vi "Read Camera Setup.vi"(8 "error in (no error)":errorcluster, 10 "String Camera Setup":string="Acquisition Mode // 1\rRead Mode // 0\rTrigger // 0\rConventional/EM // 1\rShutter Mode // 2\rShutter TTL // 0\rTime to open Shutter // 50\rTime to close Shutter // 50\rExposure time // 0\rReadout Rate // 0\rVShift Speed // 0\rPre amp // 1\rInitial line // 1\rInitial column // 1\rFinal column // 1\rFinal line // 1\rhbin // 1\rvbin // 1\rTemperature // 20\rCooler ON/OFF // 0\rFITS Format // 0\rtiff position // 1\rTiff Type // 0\rImage Format // 0\r", 11 "Construct String Setup Cam in":refnum<class "Construct String Setup Cam.lvclass">) -> (0 "error out":errorcluster, 2 "Camera Setup":T1={"Acquisition Mode"=1, "Read Mode"=4, "Trigger"=0, "Conventional/EM"=0, "Shutter Mode"=2, "Shutter TTL"=0, "Time to open Shutter"=50, "Time to close Shutter"=50, "Exposure time"=0.0, "Readout Rate"=0, "VShift Speed"=0, "Pre amp"=0, "Initial line"=1, "Initial column"=1, "Final column"=1024, "Final line"=1024, "hbin"=1, "vbin"=1, "Temperature"=20.0, "Cooler ON/OFF"=0, "FITS Format"=0, "tiff position"=1, "Tiff Type"=0, "Image Format"="", "Image Path"=""} {"Tiff Type" items=["8-bit", "16-bit", "Color"]; "FITS Format" items=["Unsigned 16", "Unsigned 32", "Signed 16", "Signed 32", "Float"]; "Cooler ON/OFF" items=["Cooler OFF", "Cooler ON"]; "Shutter TTL" items=["TTL Low", "TTL High"]; "Shutter Mode" items=["Fully Auto", "OPEN", "CLOSED"]; "Conventional/EM" items=["Conventional", "EM Gain"]; "Trigger" items=["Internal", "External", "N/A", "N/A", "N/A", "N/A", "External Start", "External Exposure (bulb)", "N/A", "External FVB EM", "Software", "N/A", "External Charge Shifting"]; "Read Mode" items=["Full Vertical Binning", "Multi-Track", "Random-Track", "Single-Track", "Image"]; "Acquisition Mode" items=["RESERVED", "Single Scan", "Accumulate", "Kinetics", "Fast Kinetics", "Run Til Abort", "RESERVED", "RESERVED", "RESERVED", "RESERVED", "Time Delayed Integration"]}, 3 "Construct String Setup Cam out":refnum<class "Construct String Setup Cam.lvclass">)   [LabVIEW 2018, in "Construct String Setup Cam.lvclass"]
doc: "Este VI recebe uma string contendo a configuração da câmera e retorna um cluster com as informações da configuração."
uses:
  Construct String Setup Cam.lvclass
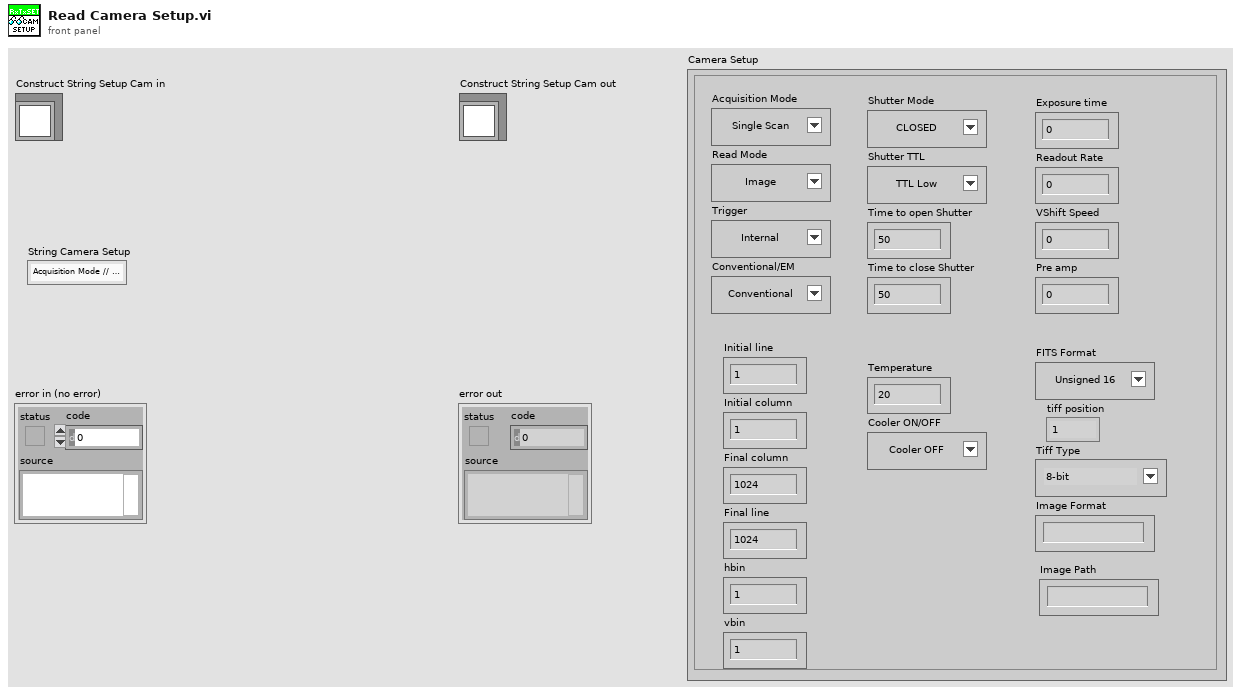
[diagram p1: front panel]
types:
  T1 = cluster{"Acquisition Mode":u16, "Read Mode":u16, "Trigger":u16, "Conventional/EM":u16, "Shutter Mode":u16, "Shutter TTL":u16, "Time to open Shutter":u16, "Time to close Shutter":u16, "Exposure time":dbl, "Readout Rate":u16, "VShift Speed":u16, "Pre amp":u16, "Initial line":u16, "Initial column":u16, "Final column":u32, "Final line":u32, "hbin":u16, "vbin":u16, "Temperature":dbl, "Cooler ON/OFF":u16, "FITS Format":u16, "tiff position":u16, "Tiff Type":u16, "Image Format":string, "Image Path":string}
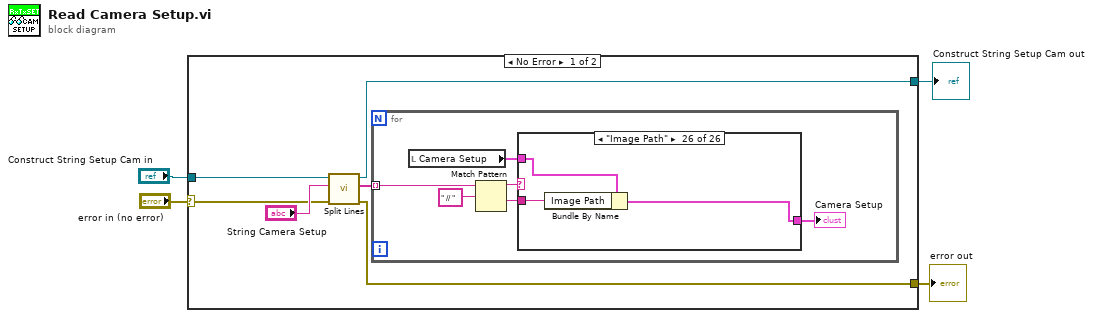
[diagram p0: block diagram]
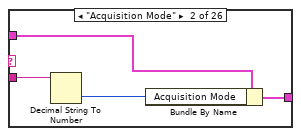
[diagram p3: hidden frame]
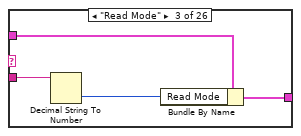
[diagram p4: hidden frame]
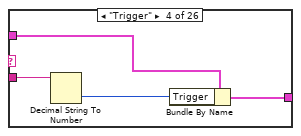
[diagram p5: hidden frame]
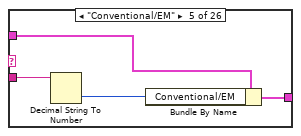
[diagram p6: hidden frame]
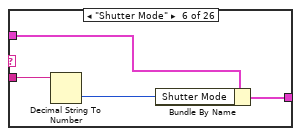
[diagram p7: hidden frame]
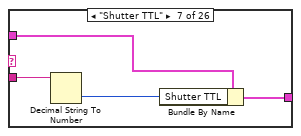
[diagram p8: hidden frame]
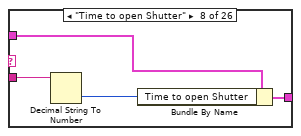
[diagram p9: hidden frame]
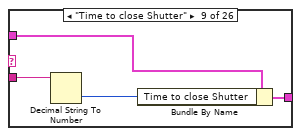
[diagram p10: hidden frame]
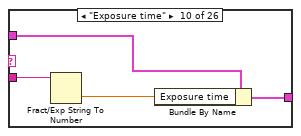
[diagram p11: hidden frame]
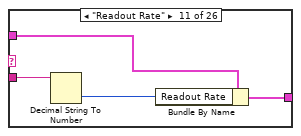
[diagram p12: hidden frame]
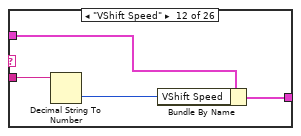
[diagram p13: hidden frame]
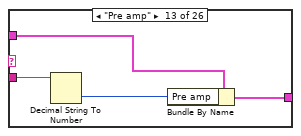
[diagram p14: hidden frame]
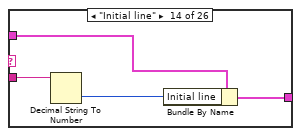
[diagram p15: hidden frame]
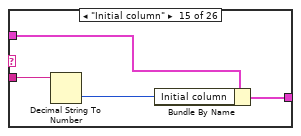
[diagram p16: hidden frame]
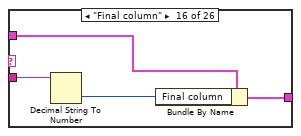
[diagram p17: hidden frame]
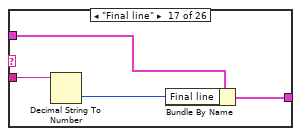
[diagram p18: hidden frame]
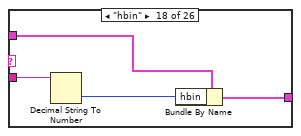
[diagram p19: hidden frame]
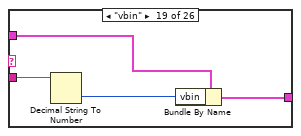
[diagram p20: hidden frame]
diagram:
  n1 = case shown="No Error" "error in (no error)" {
    selector: "error in (no error)" -> [w9 w116]
    tunnel: [w8 w116] -> w3
    tunnel: [w6 w117] -> w1
    tunnel: "Construct String Setup Cam in" -> [w7 w117]
    frame No Error {
      n2 = call "Split Lines.vi"("error in (no error)"=w9, "spreadsheet string"="String Camera Setup", "Construct String Setup Cam in"=w7) -> ("error out"=w8:errorcluster, "array"=w5:string[], "Construct String Setup Cam out"=w6:refnum<class "Construct String Setup Cam.lvclass">)  [unwired: 6 in]
      n3 = for {
        tunnel: w5 -> [w16] mode=indexing
        n4 = local read "Camera Setup"() -> (w12:T1)
        n5 = Match Pattern(string=w16, regular expression=" // ") -> (before substring=w14:string, after substring=w13:string)  [unwired: 1 in, 2 out]
        n6 = case shown="\"Image Path\"" w14 {
          tunnel: w13 -> [_ w19 w22 w26 w30 w34 w38 w42 w46 w50 w54 w58 w62 w66 w70 w74 w78 w82 w86 w90 w94 w98 w102 w106 w110 w113]
          tunnel: w12 -> [w17 w21 w24 w28 w32 w36 w40 w44 w48 w52 w56 w60 w64 w68 w72 w76 w80 w84 w88 w93 w96 w100 w104 w108 w112 w115]
          tunnel: [w17 w20 w23 w27 w31 w35 w39 w43 w47 w51 w55 w59 w63 w67 w71 w75 w79 w83 w87 w92 w95 w99 w103 w107 w111 w114] -> w11
          frame "False", Default {
          }
          frame "Acquisition Mode" {
            n7 = Decimal String To Number(string=w19) -> (number=w18:i32)  [unwired: 2 in, 1 out]
            n8 = Bundle By Name(cluster=w21, "Acquisition Mode"=w18) -> (w20:T1)
          }
          frame "Read Mode" {
            n9 = Decimal String To Number(string=w22) -> (number=w25:i32)  [unwired: 2 in, 1 out]
            n10 = Bundle By Name(cluster=w24, "Read Mode"=w25) -> (w23:T1)
          }
          frame "Trigger" {
            n11 = Decimal String To Number(string=w26) -> (number=w29:i32)  [unwired: 2 in, 1 out]
            n12 = Bundle By Name(cluster=w28, "Trigger"=w29) -> (w27:T1)
          }
          frame "Conventional/EM" {
            n13 = Decimal String To Number(string=w30) -> (number=w33:i32)  [unwired: 2 in, 1 out]
            n14 = Bundle By Name(cluster=w32, "Conventional/EM"=w33) -> (w31:T1)
          }
          frame "Shutter Mode" {
            n15 = Decimal String To Number(string=w34) -> (number=w37:i32)  [unwired: 2 in, 1 out]
            n16 = Bundle By Name(cluster=w36, "Shutter Mode"=w37) -> (w35:T1)
          }
          frame "Shutter TTL" {
            n17 = Decimal String To Number(string=w38) -> (number=w41:i32)  [unwired: 2 in, 1 out]
            n18 = Bundle By Name(cluster=w40, "Shutter TTL"=w41) -> (w39:T1)
          }
          frame "Time to open Shutter" {
            n19 = Decimal String To Number(string=w42) -> (number=w45:i32)  [unwired: 2 in, 1 out]
            n20 = Bundle By Name(cluster=w44, "Time to open Shutter"=w45) -> (w43:T1)
          }
          frame "Time to close Shutter" {
            n21 = Decimal String To Number(string=w46) -> (number=w49:i32)  [unwired: 2 in, 1 out]
            n22 = Bundle By Name(cluster=w48, "Time to close Shutter"=w49) -> (w47:T1)
          }
          frame "Exposure time" {
            n23 = Fract/Exp String To Number(string=w50) -> (number=w53:dbl)  [unwired: 3 in, 1 out]
            n24 = Bundle By Name(cluster=w52, "Exposure time"=w53) -> (w51:T1)
          }
          frame "Readout Rate" {
            n25 = Decimal String To Number(string=w54) -> (number=w57:i32)  [unwired: 2 in, 1 out]
            n26 = Bundle By Name(cluster=w56, "Readout Rate"=w57) -> (w55:T1)
          }
          frame "VShift Speed" {
            n27 = Decimal String To Number(string=w58) -> (number=w61:i32)  [unwired: 2 in, 1 out]
            n28 = Bundle By Name(cluster=w60, "VShift Speed"=w61) -> (w59:T1)
          }
          frame "Pre amp" {
            n29 = Decimal String To Number(string=w62) -> (number=w65:i32)  [unwired: 2 in, 1 out]
            n30 = Bundle By Name(cluster=w64, "Pre amp"=w65) -> (w63:T1)
          }
          frame "Initial line" {
            n31 = Decimal String To Number(string=w66) -> (number=w69:i32)  [unwired: 2 in, 1 out]
            n32 = Bundle By Name(cluster=w68, "Initial line"=w69) -> (w67:T1)
          }
          frame "Initial column" {
            n33 = Decimal String To Number(string=w70) -> (number=w73:i32)  [unwired: 2 in, 1 out]
            n34 = Bundle By Name(cluster=w72, "Initial column"=w73) -> (w71:T1)
          }
          frame "Final column" {
            n35 = Decimal String To Number(string=w74) -> (number=w77:i32)  [unwired: 2 in, 1 out]
            n36 = Bundle By Name(cluster=w76, "Final column"=w77) -> (w75:T1)
          }
          frame "Final line" {
            n37 = Decimal String To Number(string=w78) -> (number=w81:i32)  [unwired: 2 in, 1 out]
            n38 = Bundle By Name(cluster=w80, "Final line"=w81) -> (w79:T1)
          }
          frame "hbin" {
            n39 = Decimal String To Number(string=w82) -> (number=w85:i32)  [unwired: 2 in, 1 out]
            n40 = Bundle By Name(cluster=w84, "hbin"=w85) -> (w83:T1)
          }
          frame "vbin" {
            n41 = Decimal String To Number(string=w86) -> (number=w89:i32)  [unwired: 2 in, 1 out]
            n42 = Bundle By Name(cluster=w88, "vbin"=w89) -> (w87:T1)
          }
          frame "Temperature" {
            n43 = Fract/Exp String To Number(string=w90) -> (number=w91:dbl)  [unwired: 3 in, 1 out]
            n44 = Bundle By Name(cluster=w93, "Temperature"=w91) -> (w92:T1)
          }
          frame "Cooler ON/OFF" {
            n45 = Decimal String To Number(string=w94) -> (number=w97:i32)  [unwired: 2 in, 1 out]
            n46 = Bundle By Name(cluster=w96, "Cooler ON/OFF"=w97) -> (w95:T1)
          }
          frame "FITS Format" {
            n47 = Decimal String To Number(string=w98) -> (number=w101:i32)  [unwired: 2 in, 1 out]
            n48 = Bundle By Name(cluster=w100, "FITS Format"=w101) -> (w99:T1)
          }
          frame "tiff position" {
            n49 = Decimal String To Number(string=w102) -> (number=w105:i32)  [unwired: 2 in, 1 out]
            n50 = Bundle By Name(cluster=w104, "tiff position"=w105) -> (w103:T1)
          }
          frame "Tiff Type" {
            n51 = Decimal String To Number(string=w106) -> (number=w109:i32)  [unwired: 2 in, 1 out]
            n52 = Bundle By Name(cluster=w108, "Tiff Type"=w109) -> (w107:T1)
          }
          frame "Image Format" {
            n53 = Bundle By Name(cluster=w112, "Image Format"=w110) -> (w111:T1)
          }
          frame "Image Path" {
            n54 = Bundle By Name(cluster=w115, "Image Path"=w113) -> (w114:T1)
          }
        }
        "Camera Setup" <- w11
      }
    }
    frame Error {
    }
  }
  "error out" <- w3
  "Construct String Setup Cam out" <- w1
